vi "Camera-DeviceClear.vi"(0 "Camera Device OUT":T1) -> ()   [LabVIEW 2010]
uses:
  <vilib>/Utility/error.llb/DialogType.ctl
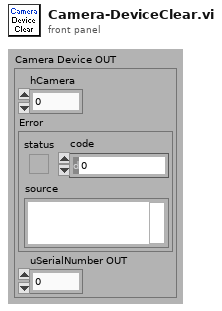
[diagram p1: front panel]
types:
  T1 = cluster{"hCamera":u32, "Error":errorcluster, "uSerialNumber OUT":u32}
  T2 = typedef "DialogType.ctl" = u16
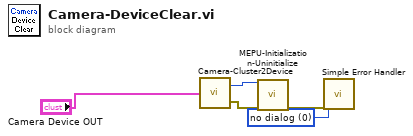
[diagram p0: block diagram]
diagram:
  w5 = T2 0 items=["no dialog", "OK message", "continue or stop message", "OK message + warnings", "continue/stop + warnings"] ("type of dialog (OK msg:1)")
  n1 = call "Camera-Cluster2Device.vi"("Camera Device IN"="Camera Device OUT") -> ("Error OUT"=w2:errorcluster, "hCamera OUT"=w1:u32)  [unwired: 2 in, 1 out]
  n2 = call <vilib>:"MEPU-Initialization-Uninitialize.vi"("hCamera IN"=w1, "Error IN"=w2) -> ("Error OUT"=w4:errorcluster)  [unwired: 13 in]
  n3 = call <vilib>:"Simple Error Handler.vi"("type of dialog (OK msg:1)"=w5, "error in (no error)"=w4) -> ()  [unwired: 3 in, 5 out]
